vi "ProcessUDPValues.vi"(8 "error in (no error)":errorcluster, 11 "connection ID":refnum<k16>) -> ()   [LabVIEW 2015]
uses:
  GlobalVisionVars.vi
panel:
  out "ProcessTime":dbl
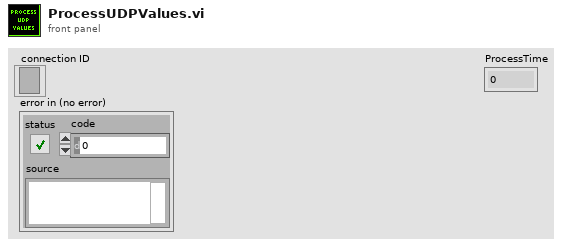
[diagram p1: front panel]
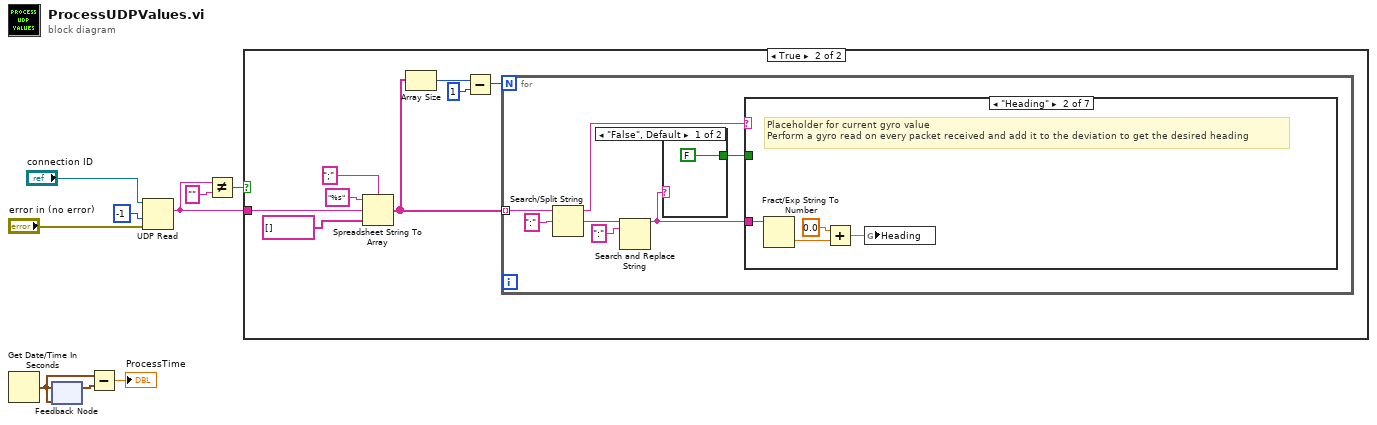
[diagram p0: block diagram]
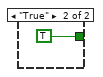
[diagram p3: hidden frame]
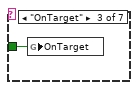
[diagram p5: hidden frame]
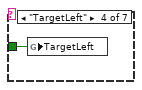
[diagram p6: hidden frame]
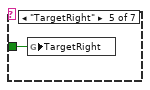
[diagram p7: hidden frame]
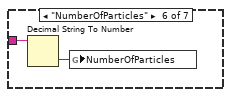
[diagram p8: hidden frame]
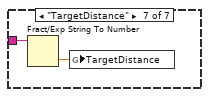
[diagram p9: hidden frame]
diagram:
  n1 = Get Date/Time In Seconds() -> (seconds since 1Jan1904=w7:timestamp)
  n2 = feedback-in #1(w7) -> ()
  n3 = feedback #1(w7) -> (w9:timestamp)
  n4 = Subtract(x=w7, y=w9) -> (x-y=→"ProcessTime":dbl)
  n5 = UDP Read(connection ID="connection ID", timeout ms (25000)=-1, 8:"error in (no error)") -> (data out=w1:string)  [unwired: 1 in, 4 out]
  n6 = Not Equal?(x=w1, y="") -> (x != y?=w2:bool)
  n7 = case shown="True" w2 {
    tunnel: w1 -> [_ w17]
    frame False {
    }
    frame True {
      n8 = Spreadsheet String To Array(delimiter (Tab)=";" ("search string/char (-)"), format string="%s", spreadsheet string=w17, array type (2D Dbl)=string[] []) -> (array=w13:string[])
      n9 = Array Size(array=w13) -> (size(s)=w12:i32)
      n10 = Subtract(x=w12, y=1) -> (x-y=w10:i32)
      n11 = for {
        N: w10 -> [_]
        tunnel: w13 -> [w24] mode=indexing
        n12 = Search/Split String(string=w24, search string/char (-)=":") -> (substring before match=w22:string, match + rest of string=w21:string)  [unwired: 1 in, 1 out]
        n13 = Search and Replace String(input string=w21, search string=":" ("replace string (\"\")")) -> (result string=w19:string)  [unwired: 6 in, 3 out]
        n14 = case shown="\"False\", Default" w19 {
          tunnel: [FALSE TRUE] -> w18
          frame "False", Default {
          }
          frame "True" {
          }
        }
        n15 = case shown="\"Heading\"" w22 {
          tunnel: w19 -> [_ w30 _ _ _ w35 w36]
          tunnel: w18 -> [_ _ w31 w32 w33 _ _]
          frame "False", Default {
          }
          frame "Heading" {
            # "Placeholder for current gyro value\nPerform a gyro read on every packet received and add it to the deviation to get the desired heading"
            n16 = Fract/Exp String To Number(string=w30) -> (number=w28:dbl)  [unwired: 3 in, 1 out]
            n17 = Add(x=0.0, y=w28) -> (x+y=w29:dbl)
            n18 = global write "GlobalVisionVars.vi" "Heading"(w29) -> ()
          }
          frame "OnTarget" {
            n19 = global write "GlobalVisionVars.vi" "OnTarget"(w31) -> ()
          }
          frame "TargetLeft" {
            n20 = global write "GlobalVisionVars.vi" "TargetLeft"(w32) -> ()
          }
          frame "TargetRight" {
            n21 = global write "GlobalVisionVars.vi" "TargetRight"(w33) -> ()
          }
          frame "NumberOfParticles" {
            n22 = Decimal String To Number(string=w35) -> (number=w34:i32)  [unwired: 2 in, 1 out]
            n23 = global write "GlobalVisionVars.vi" "NumberOfParticles"(w34) -> ()
          }
          frame "TargetDistance" {
            n24 = Fract/Exp String To Number(string=w36) -> (number=w37:dbl)  [unwired: 3 in, 1 out]
            n25 = global write "GlobalVisionVars.vi" "TargetDistance"(w37) -> ()
          }
        }
      }
    }
  }
